vi "AckNack Response.vi"(8 "error in (no error)":errorcluster, 9 "Original TCP Payload":T2, 10 "Result":T1=enum."RESULT_UNKNOWN", 11 "TCPMessageService in":refnum<class "TCPMessageAPI.lvclass">) -> (0 "error out":errorcluster, 3 "TCPMessageService out":refnum<class "TCPMessageAPI.lvclass">)   [LabVIEW 2020, in "Vecto.lvlib" / "TCPMessageAPI.lvclass"]
uses:
  TCPMessageAPI.lvclass
  proto/TcpPayload/Data.ctl
  proto/AckNackResult/Enumeration.ctl
  proto/TcpAckNack/Data.ctl
  proto/AckNackResult/AckNackResult.lvlib
  proto/TcpAckNack/TcpAckNack.lvlib
  proto/TcpPayload/TcpPayload.lvlib
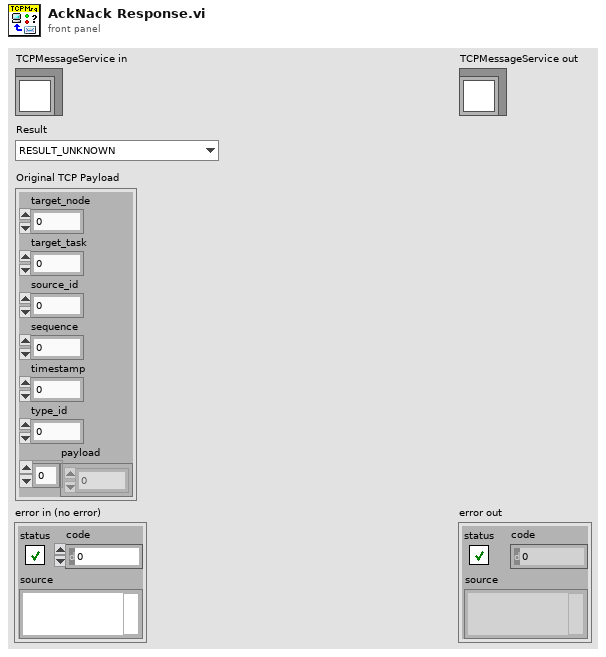
[diagram p1: front panel]
types:
  T1 = typedef "AckNackResult.lvlib/Enumeration.ctl" = enum16{"RESULT_PAYLOAD_ERROR", "RESULT_UNEXPECTED_TYPE", "RESULT_EXPIRED", "RESULT_OUTOFSEQUENCE", "RESULT_DISALLOWED", "RESULT_INVALIDTASK", "RESULT_INVALIDTARGET", "RESULT_UNKNOWN", "RESULT_ACK"}
  T2 = typedef "TcpPayload.lvlib/Data.ctl" = cluster{"target_node":u32, "target_task":u32, "source_id":u32, "sequence":u32, "timestamp":u64, "type_id":u32, "payload":u8[]}
  T3 = typedef "TcpAckNack.lvlib/Data.ctl" = cluster{"target_node":u32, "target_task":u32, "sequence":u32, "timestamp":u64, "type_id":u32, "result":T1}
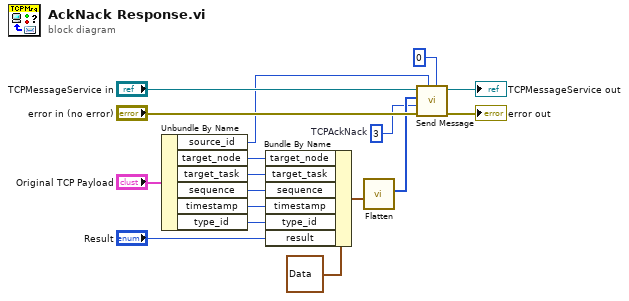
[diagram p0: block diagram]
diagram:
  w4 = u32 3  # TCPAckNack
  n1 = Unbundle By Name("Original TCP Payload") -> ("source_id"=w5:u32, "target_node"=w12:u32, "target_task"=w11:u32, "sequence"=w10:u32, "timestamp"=w9:u64, "type_id"=w7:u32)
  n2 = Bundle By Name(cluster=T3 {"target_node"=0, "target_task"=0, "sequence"=0, "timestamp"=0, "type_id"=0, "result"=enum."RESULT_UNKNOWN"} ("TcpNack"), "target_node"=w12, "target_task"=w11, "sequence"=w10, "timestamp"=w9, "type_id"=w7, "result"="Result") -> (w8:T3)
  n3 = call "Flatten.vi"("Data"=w8) -> ("Buffer"=w6:u8[])  [unwired: 9 in, 1 out]
  n4 = call "Send Message.vi"("Target Task"=u32 0, "Target Node"=w5, "error in (no error)"="error in (no error)", "Type ID"=w4, "Payload"=w6, "TCPMessageService in"="TCPMessageService in") -> ("error out"=→"error out":errorcluster, "TCPMessageService out"=→"TCPMessageService out":refnum<class "TCPMessageAPI.lvclass">)  [unwired: 4 in]
